vi "change_voltages_in_process_list.vi"(0 "Process list":T1, 1 "iteration number":i32, 3 "Variable Steps":bool, 4 "Num files":i32=1) -> (2 "output process list":T1)   [LabVIEW 2018]
panel:
  in  "Process list 2":T1
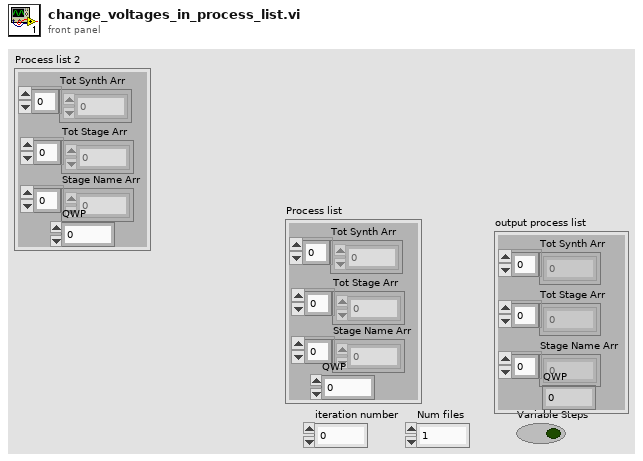
[diagram p1: front panel]
types:
  T1 = cluster{"Tot Synth Arr":dbl[], "Tot Stage Arr":dbl[], "Stage Name Arr":dbl[], "QWP":dbl}
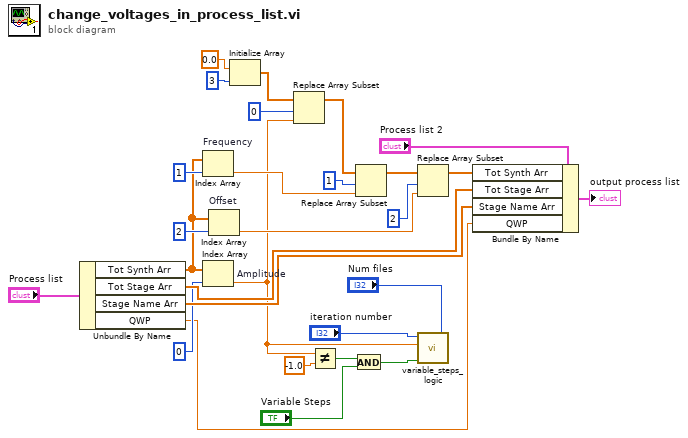
[diagram p0: block diagram]
diagram:
  n1 = Unbundle By Name("Process list") -> ("Tot Synth Arr"=w19:dbl[], "Tot Stage Arr"=w26:dbl[], "Stage Name Arr"=w25:dbl[], "QWP"=w1:dbl)
  n2 = Index Array "Frequency"(array=w19, index=1) -> (element=w12:dbl)
  n3 = Index Array "Amplitude"(array=w19, index=0) -> (element=w2:dbl)
  n4 = Index Array "Offset"(array=w19, index=2) -> (element=w11:dbl)
  n5 = Initialize Array(0.0 ("element"), 3 ("dimension size")) -> (w15:dbl[])
  n6 = Replace Array Subset(array=w15, new element=w2, index=0 ("x+y")) -> (w17:dbl[])
  n7 = Not Equal?(x=w2, y=-1.0) -> (x != y?=w6:bool)
  n8 = And(x=w6, y="Variable Steps") -> (x .and. y?=w4:bool)
  n9 = Replace Array Subset(array=w17, new element=w12, index=1 ("disabled index (col)")) -> (w16:dbl[])
  n10 = Replace Array Subset(array=w16, new element=w11, index=2 ("disabled index (col)")) -> (w8:dbl[])
  n11 = call "variable_steps_logic.vi"("Num files"="Num files", "Variable Steps"=w4, "Voltage 1"=w2, "iteration number"="iteration number") -> ()  [unwired: 1 in, 2 out]
  n12 = Bundle By Name(cluster="Process list 2", "Tot Synth Arr"=w8, "Tot Stage Arr"=w26, "Stage Name Arr"=w25, "QWP"=w1) -> (→"output process list":T1)
